vi "SwerveDriveSafetyTest.vi"   [LabVIEW 2019, in "Swerve Drive.lvlib"]
doc: "Calls the SafetyCheck VI. SafetyCheck VI needs to be called dynamically by the SafetyCheckEngine, but it already gets called statically. Wrapping it in this VI enables calling it dynamically."
uses:
  Swerve Drive.lvlib
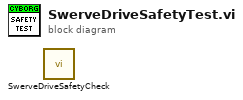
[diagram p0: block diagram]
diagram:
  n1 = call "SwerveDriveSafetyCheck.vi"() -> ()  [unwired: 15 in, 1 out]
